vi "SEA_9811_Clock_sync.vi"(8 "error in (no error)":errorcluster, 11 "SEA9811_RT_data in":T1) -> (0 "error out":errorcluster, 3 "SEA9811_RT_data out":T1)   [LabVIEW 2012]
doc: "Synchronize current RT time to FPGA timekeeper"
uses:
  Typdefs/SEA9811_RT_data_cluster.ctl
  <userlib>/_FPGA Interface Advanced Tools/FPGA Interface Base/FPGA Interface Base.lvclass
  Typdefs/FPGA ref.ctl
  Typdefs/channel.ctl
  Typdefs/received word.ctl
  Typdefs/SEA9811_FPGA_FP_Addresses.ctl
  <userlib>/_FPGA Interface Advanced Tools/FPGA Interface Wrapper/NiFPGA Write - U64.vi
  <vilib>/Utility/error.llb/Error Cluster From Error Code.vi
  <userlib>/FPGA Timekeeper 1.1b0/FPGA Timekeeper.lvlib
  <userlib>/_FPGA Interface Advanced Tools/FPGA Interface Wrapper/FPGA Interface Wrapper.lvlib
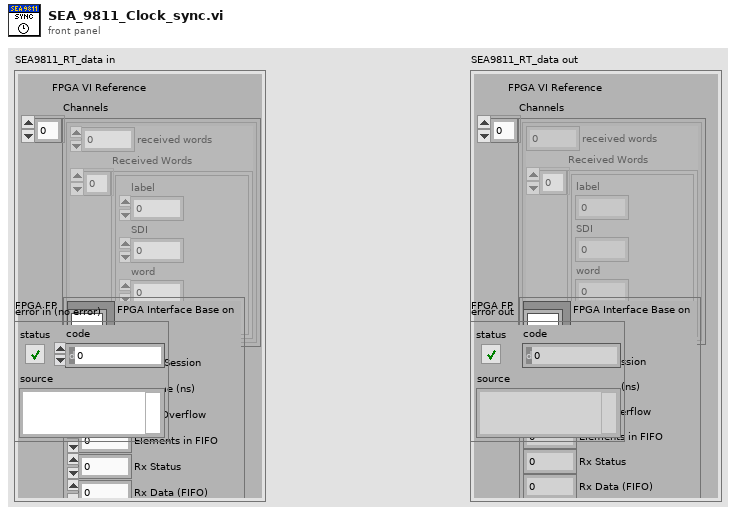
[diagram p1: front panel]
types:
  T1 = typedef "SEA9811_RT_data_cluster.ctl" = cluster{"FPGA VI Reference":T2, "Channels":T3[], "FPGA FP":T5}
  T2 = typedef "FPGA ref.ctl" = refnum<k20>
  T3 = typedef "channel.ctl" = cluster{"received words":u32, "Received Words":T4[]}
  T4 = typedef "received word.ctl" = cluster{"label":u8, "SDI":u8, "word":u32, "timestamp":dbl}
  T5 = typedef "SEA9811_FPGA_FP_Addresses.ctl" = cluster{"FPGA Interface Base on":refnum<class "FPGA Interface Base.lvclass">, "FPGA Session":u32, "RT time (ns)":u32, "DMA Overflow":u32, "Elements in FIFO":u32, "Rx Status":u32, "Rx Data (FIFO)":u32}
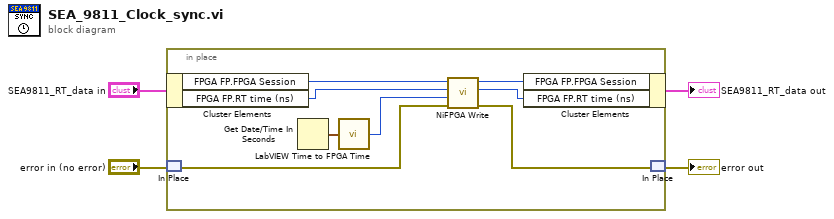
[diagram p0: block diagram]
diagram:
  n1 = in-place {
    n2 = in-place-cluster #1("SEA9811_RT_data in") -> ("FPGA FP.FPGA Session"=w11:u32, "FPGA FP.RT time (ns)"=w5:u32)
    n3 = in-place-match #2("error in (no error)") -> (w6:errorcluster)
    n4 = Get Date/Time In Seconds() -> (seconds since 1Jan1904=w10:timestamp)
    n5 = call <userlib>:"LabVIEW Time to FPGA Time.vi"("LabVIEW time"=w10) -> ("FPGA time (ns)"=w7:u64)
    n6 = call-poly <userlib>:"NiFPGA Write.vi"("error in (no error)"=w6, "Value"=w7, "Control"=w5, "Session"=w11) -> ("error out"=w8:errorcluster, "Session Out"=w9:u32)  [unwired: 6 in]
    n7 = in-place-cluster #1("FPGA FP.FPGA Session"=w9, "FPGA FP.RT time (ns)"=w5) -> (→"SEA9811_RT_data out":T1)
    n8 = in-place-match #2(w8) -> (→"error out":errorcluster)
  }
